vi "Set Instrument From Marker.vi"(8 "error in (no error)":errorcluster, 9 "Marker To (0: Center Frequency)":i32(ring) items=["Center Frequency", "Start Frequency", "Stop Frequency"], 10 "Active Marker (1: Marker 1)":i32(ring)=1 items=["Marker 1"=1, "Marker 2"=2, "Marker 3"=3, "Marker 4"=4, "Marker 5"=5, "Marker 6"=6], 11 "VISA resource name":refnum<visa-resource-name>) -> (0 "error out":errorcluster, 3 "VISA resource name out":refnum<visa-resource-name>)   [LabVIEW 2022 SP3, in "Agilent N934X Series.lvlib"]
doc: "Sets the reference level or center frequency to the value of the selected marker."
uses:
  <instrlib>/Agilent N934X Series/Agilent N934X Series.lvlib
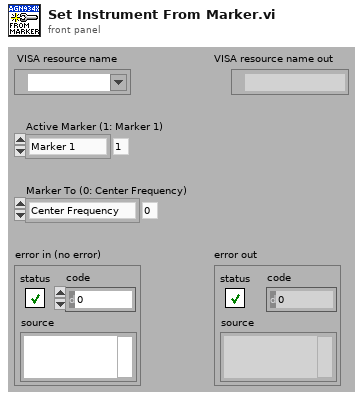
[diagram p1: front panel]
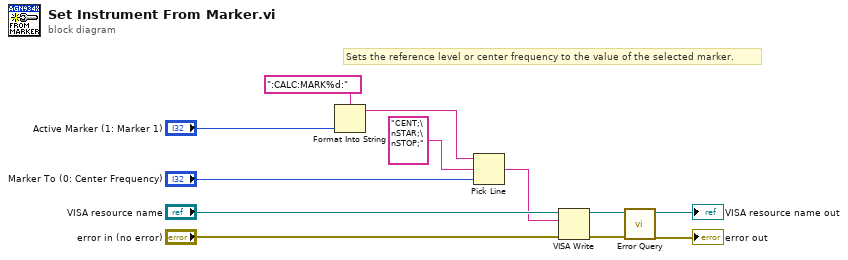
[diagram p0: block diagram]
diagram:
  # "Sets the reference level or center frequency to the value of the selected marker."
  n1 = Format Into String(format string=":CALC:MARK%d:", "Active Marker (1: Marker 1)") -> (resulting string=w3:string)  [unwired: 2 in, 1 out]
  n2 = Pick Line(string ("")=w3, multi-line string="CENT;\nSTAR;\nSTOP;", line index="Marker To (0: Center Frequency)") -> (output string=w1:string)
  n3 = VISA Write(VISA resource name="VISA resource name", write buffer=w1, error in (no error)="error in (no error)") -> (VISA resource name out=w8:refnum<visa-resource-name>, error out=w7:errorcluster)  [unwired: 1 out]
  n4 = call <instrlib>:"Error Query.vi"("error in (no error)"=w7, "VISA resource name"=w8) -> ("error out"=→"error out":errorcluster, "VISA resource name out"=→"VISA resource name out":refnum<visa-resource-name>)  [unwired: 6 in, 2 out]
